vi "Write Report.vi"(8 "error in (no error)":errorcluster, 10 "Resource In":variant, 11 "Analyze Results Fluence and Energy in":refnum<class "Analyze Results Fluence and Energy.lvclass">) -> (0 "error out":errorcluster, 2 "Resource Out":variant, 3 "Analyze Results Fluence and Energy out":refnum<class "Analyze Results Fluence and Energy.lvclass">)   [LabVIEW 2014, in "Analyze Results Fluence and Energy.lvclass"]
uses:
  Analyze Results Fluence and Energy.lvclass
  Analyze Results Fluence and Energy.lvclass/Analyze Results Fluence and Energy.ctl
  JETI200 Overview and ShotID/HIJ Vision/Analyze/Results and Overlays/Results Base/Analyze Results Base.lvclass
  JETI200 Overview and ShotID/HIJ Vision/Analyze/Results and Overlays/Results Energy/Analyze Results Energy.lvclass
  JETI200 Overview and ShotID/HIJ Vision/Analyze/Results and Overlays/Results Fluence/Analyze Results Fluence.lvclass
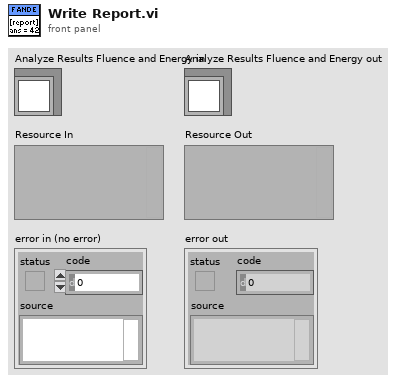
[diagram p1: front panel]
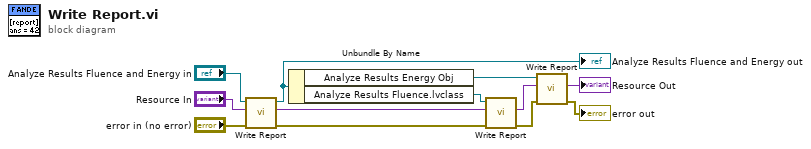
[diagram p0: block diagram]
diagram:
  n1 = call-parent "Write Report.vi"("error in (no error)"="error in (no error)", "Resource In"="Resource In", "Analyze Results Base in"="Analyze Results Fluence and Energy in") -> ("error out"=w3:errorcluster, "Resource Out"=w4:variant, "Analyze Results Base out"=w9:refnum<class "Analyze Results Fluence and Energy.lvclass">)  [unwired: 6 in]
  "Analyze Results Fluence and Energy out" <- w9
  n2 = Unbundle By Name(w9) -> ("Analyze Results Energy Obj"=w8:refnum<class "Analyze Results Energy.lvclass">, "Analyze Results Fluence.lvclass"=w5:refnum<class "Analyze Results Fluence.lvclass">)
  n3 = call-dynamic "Write Report.vi"("error in (no error)"=w3, "Resource In"=w4, "Analyze Results Fluence in"=w5) -> ("error out"=w2:errorcluster, "Resource Out"=w1:variant)  [unwired: 6 in, 1 out]
  n4 = call-dynamic "Write Report.vi"("error in (no error)"=w2, "Resource In"=w1, "Analyze Results Energy in"=w8) -> ("error out"=→"error out":errorcluster, "Resource Out"=→"Resource Out":variant)  [unwired: 6 in, 1 out]
